vi "[CS] [Frame] Save to File.vi"(8 "array":dbl[][](array[numeric]), 10 "Name":string, 11 "base path":path) -> ()   [LabVIEW 2014]
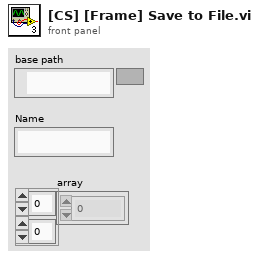
[diagram p1: front panel]
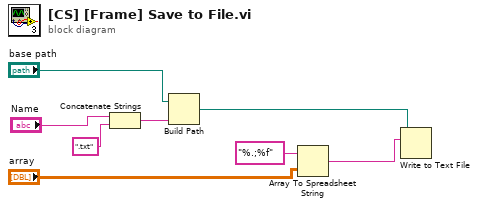
[diagram p0: block diagram]
diagram:
  n1 = Concatenate Strings("Name", ".txt" ("string")) -> (w3:string)
  n2 = Build Path(base path="base path", name or relative path=w3) -> (appended path=w5:path)
  n3 = Array To Spreadsheet String(array="array", 3:"%.;%f" ("format string")) -> (spreadsheet string=w7:string)  [unwired: 1 in]
  n4 = Write to Text File(file (use dialog)=w5, text=w7) -> ()  [unwired: 2 in, 3 out]
